vi "Transfer Multiple.vi"(5 "To Bindings":refnum<class "Binding.lvclass">[](array[class]), 7 "From Bindings":refnum<class "Binding.lvclass">[](array[class]), 8 "error in (no error)":errorcluster, 9 "To Class in":refnum<class>, 10 "From Class in":refnum<class>) -> (0 "error out":errorcluster, 1 "To Class out":refnum<class>, 2 "From Class out":refnum<class>)   [LabVIEW 2020, in "PropertyBinder.lvlib" / "Binding.lvclass"]
uses:
  Binding/Binding.lvclass
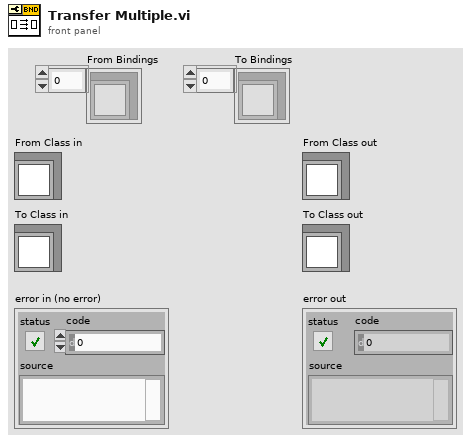
[diagram p1: front panel]
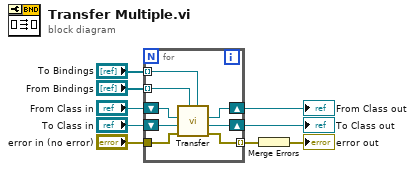
[diagram p0: block diagram]
diagram:
  n1 = for {
    shift-right: [w14] -> w3
    shift-left: "From Class in" -> [w17]
    shift-right: [w10] -> w2
    shift-left: "To Class in" -> [w13]
    tunnel: "error in (no error)" -> [w12]
    tunnel: "From Bindings" -> [w16] mode=indexing
    tunnel: "To Bindings" -> [w15] mode=indexing
    tunnel: [w11] -> w4 mode=indexing
    n2 = call "Transfer.vi"("To Binding"=w15, "From Binding"=w16, "error in (no error)"=w12, "To Class in"=w13, "From Class in"=w17) -> ("error out"=w11:errorcluster, "To Class out"=w10:refnum<class>, "From Class out"=w14:refnum<class>)  [unwired: 4 in]
  }
  "From Class out" <- w3
  "To Class out" <- w2
  n3 = Merge Errors(w4) -> (→"error out":errorcluster)
